vi "LDO Bit Status Write.vi"(8 "error in":errorcluster, 11 "LDO Control Input":T1) -> (0 "error out":errorcluster, 3 "Bit Status":string[][](array[string]))   [LabVIEW 2020]
uses:
  Modbus/Modbus LDO Control.ctl
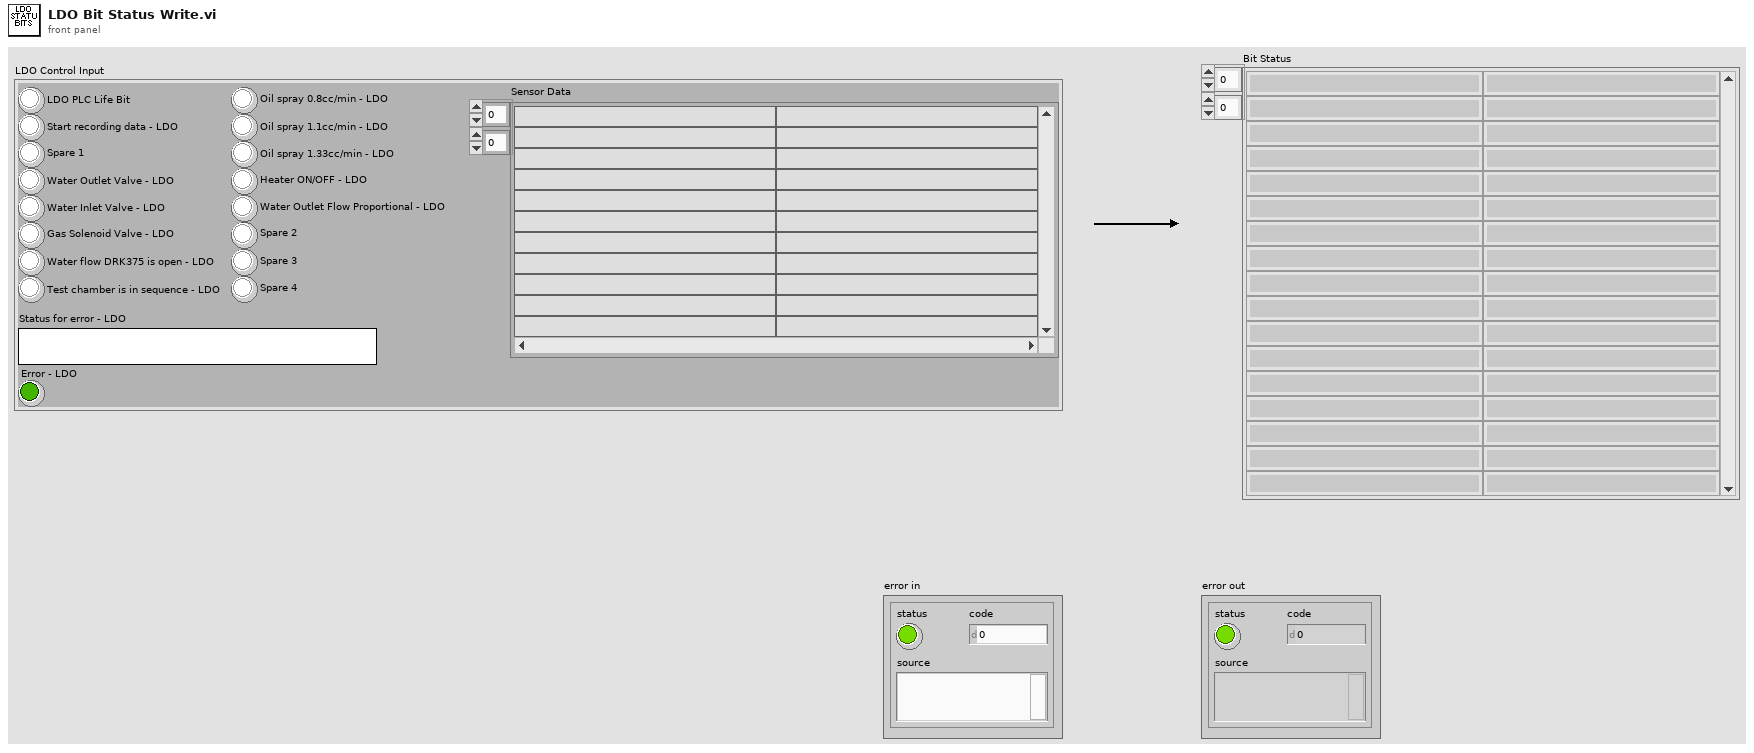
[diagram p1: front panel]
types:
  T1 = typedef "Modbus LDO Control.ctl" = cluster{"LDO PLC Life Bit":bool, "Start recording data - LDO":bool, "Spare 1":bool, "Water Outlet Valve - LDO":bool, "Water Inlet Valve - LDO":bool, "Gas Solenoid Valve - LDO":bool, "Water flow DRK375 is open - LDO":bool, "Test chamber is in sequence - LDO":bool, "Oil spray 0.8cc/min - LDO":bool, "Oil spray 1.1cc/min - LDO":bool, "Oil spray 1.33cc/min - LDO":bool, "Heater ON/OFF - LDO":bool, "Water Outlet Flow Proportional - LDO":bool, "Spare 2":bool, "Spare 3":bool, "Spare 4":bool, "Status for error - LDO":string, "Error - LDO":bool, "Sensor Data":string[][]}
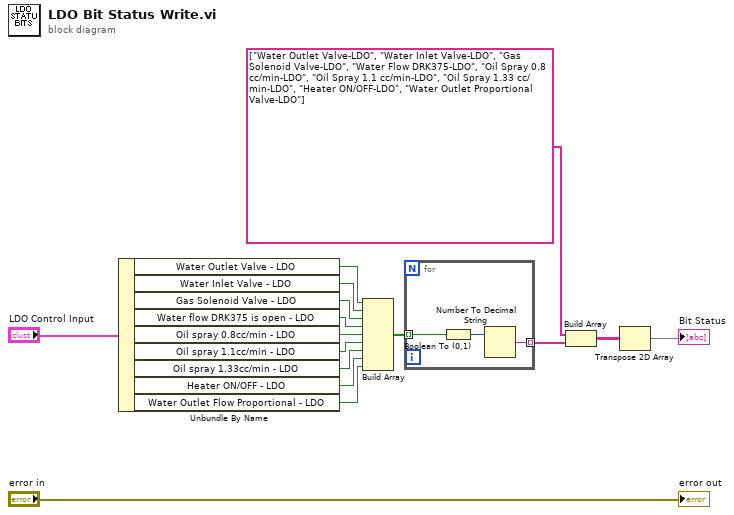
[diagram p0: block diagram]
diagram:
  n1 = Unbundle By Name("LDO Control Input") -> ("Water Outlet Valve - LDO"=w15:bool, "Water Inlet Valve - LDO"=w14:bool, "Gas Solenoid Valve - LDO"=w13:bool, "Water flow DRK375 is open - LDO"=w12:bool, "Oil spray 0.8cc/min - LDO"=w11:bool, "Oil spray 1.1cc/min - LDO"=w10:bool, "Oil spray 1.33cc/min - LDO"=w9:bool, "Heater ON/OFF - LDO"=w8:bool, "Water Outlet Flow Proportional - LDO"=w7:bool)
  n2 = Build Array(w15, w14, w13, w12, w11, w10, w9, w8, w7) -> (w6:bool[])
  n3 = for {
    tunnel: w6 -> [w18] mode=indexing
    tunnel: [w17] -> w5 mode=indexing
    n4 = Boolean To (0,1)(Boolean=w18) -> (0, 1=w19:i16)
    n5 = Number To Decimal String(number=w19) -> (decimal integer string=w17:string)  [unwired: 1 in]
  }
  n6 = Build Array(string[] ["Water Outlet Valve-LDO", "Water Inlet Valve-LDO", "Gas Solenoid Valve-LDO", "Water Flow DRK375-LDO", "Oil Spray 0.8 cc/min-LDO", "Oil Spray 1.1 cc/min-LDO", "Oil Spray 1.33 cc/min-LDO", "Heater ON/OFF-LDO", "Water Outlet Proportional Valve-LDO"], w5) -> (w3:string[][])
  n7 = Transpose 2D Array(2D array=w3) -> (transposed array=→"Bit Status":string[][])
  "error out" <- "error in"
